vi "Excute.vi"(8 "error in (no error)":errorcluster, 11 "Cmd1 in":refnum<class "Cmd1.lvclass">) -> (0 "error out":errorcluster, 3 "Cmd1 out":refnum<class "Cmd1.lvclass">)   [LabVIEW 2014, in "Cmd1.lvclass"]
uses:
  Cmd1.lvclass
  Cmd1.lvclass/Cmd1.ctl
  Worker1/Worker1(receiver).lvclass
  Worker2/Worker2(receiver).lvclass
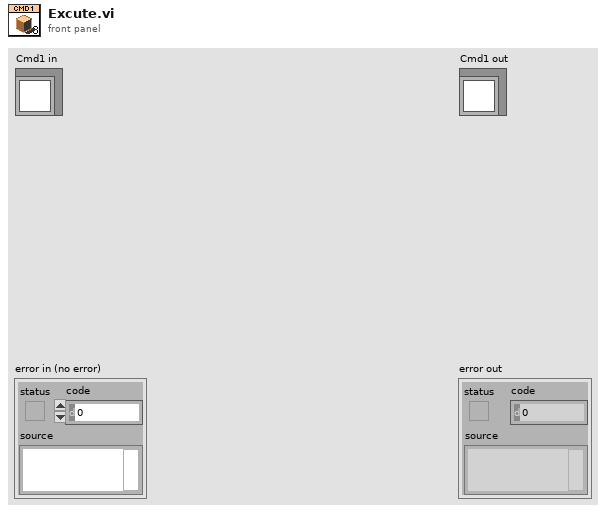
[diagram p1: front panel]
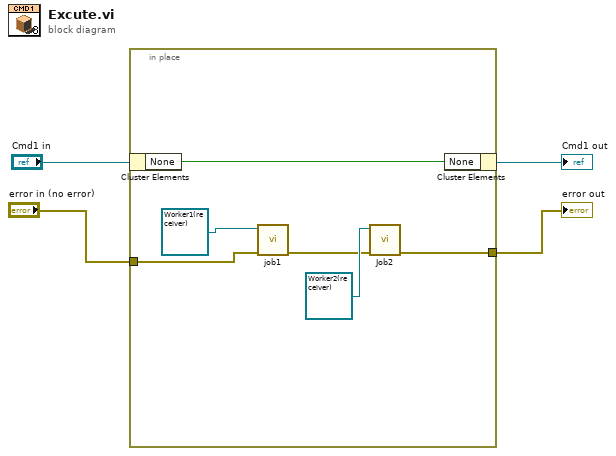
[diagram p0: block diagram]
diagram:
  n1 = in-place {
    in-place-border: "error in (no error)" -> [w6]
    in-place-border: [w5] -> w1
    n2 = in-place-cluster #1("Cmd1 in") -> ("None"=w10:bool)
    n3 = call "job1.vi"("error in (no error)"=w6, "Worker1(receiver) in"=refnum<class "Worker1(receiver).lvclass"> refnum ("Worker1(receiver).lvclass")) -> ("error out"=w7:errorcluster)  [unwired: 8 in, 1 out]
    n4 = call "Job2.vi"("error in (no error)"=w7, "Worker2(receiver) in"=refnum<class "Worker2(receiver).lvclass"> refnum ("Worker2(receiver).lvclass")) -> ("error out"=w5:errorcluster)  [unwired: 8 in, 1 out]
    n5 = in-place-cluster #1("None"=w10) -> (→"Cmd1 out":refnum<class "Cmd1.lvclass">)
  }
  "error out" <- w1
